vi "Read Workspace Manager.vi"(8 "error in (no error)":errorcluster, 11 "SLSC EDS System Tests in":refnum<class "SLSC EDS System Tests.lvclass">) -> (0 "error out":errorcluster, 2 "WorkspaceManager out":T1, 3 "SLSC EDS System Tests out":refnum<class "SLSC EDS System Tests.lvclass">)   [LabVIEW 2015, in "SLSC EDS System Tests.lvclass"]
uses:
  SLSC EDS System Tests.lvclass
  <vilib>/NI Veristand/Execution/Workspace/WorkspaceAPI.ctl
  NationalInstruments.VeriStand.ClientAPI
  SLSC EDS System Tests.lvclass/SLSC EDS System Tests.ctl
  rzoeller-veristandtestcase/VeriStand Test Utilities/VeriStand Test Utilities.lvclass
  <vilib>/NI VeriStand/Execution/Workspace/NI_VS Workspace ExecutionAPI.lvlib
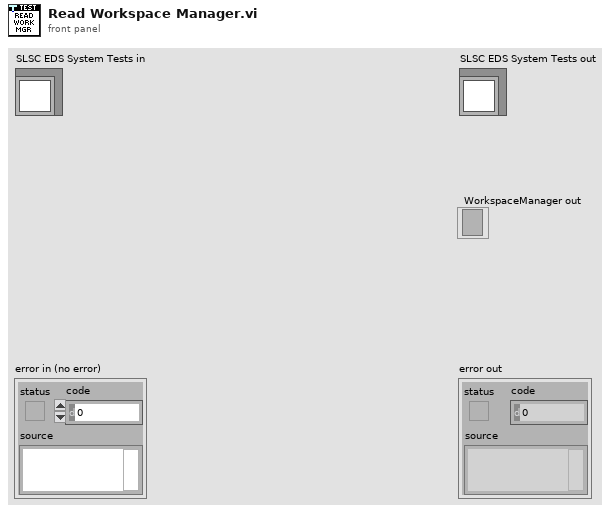
[diagram p1: front panel]
types:
  T1 = typedef "NI_VS Workspace ExecutionAPI.lvlib/WorkspaceAPI.ctl" = refnum<k24>
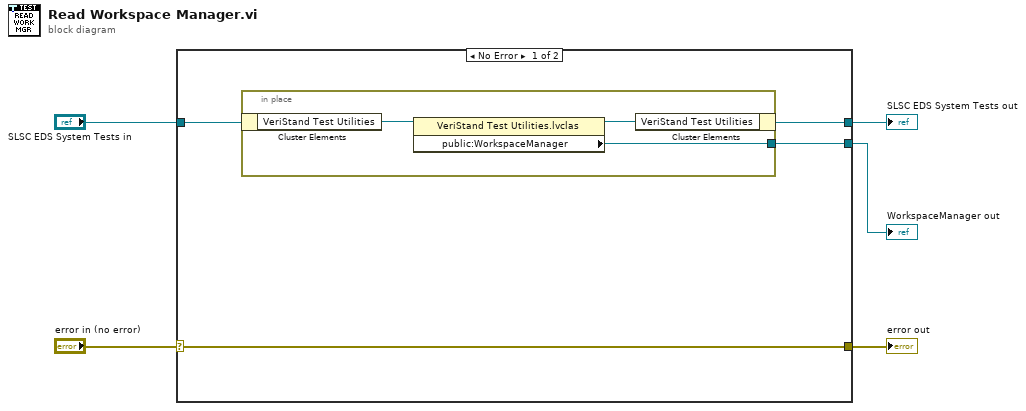
[diagram p0: block diagram]
diagram:
  n1 = case shown="No Error" "error in (no error)" {
    selector: "error in (no error)" -> [w9 w14]
    tunnel: [w9 w14] -> w4
    tunnel: [w7 w13] -> w2
    tunnel: "SLSC EDS System Tests in" -> [w8 w13]
    tunnel: [w6 _] -> w1
    frame No Error {
      n2 = in-place {
        in-place-border: [w10] -> w6
        n3 = in-place-cluster #1(w8) -> ("VeriStand Test Utilities"=w12:refnum<class "VeriStand Test Utilities.lvclass">)
        n4 = property class="VeriStand Test Utilities.lvclas"(reference=w12) -> (reference out=w11:refnum<class "VeriStand Test Utilities.lvclass">, "public:WorkspaceManager"=w10:T1)  [unwired: 1 in, 1 out]
        n5 = in-place-cluster #1("VeriStand Test Utilities"=w11) -> (w7:refnum<class "SLSC EDS System Tests.lvclass">)
      }
    }
    frame Error {
    }
  }
  "error out" <- w4
  "SLSC EDS System Tests out" <- w2
  "WorkspaceManager out" <- w1
